vi "B_WriteAttribute.vi"(0 "reference in":refnum<class "BaseTemplate.lvclass">, 5 "error in (no error)":errorcluster) -> (14 "reference out":refnum<class "BaseTemplate.lvclass">, 19 "error out":errorcluster)   [LabVIEW 2020, in "BaseTemplate.lvclass"]
uses:
  <resource>/Framework/Providers/Open_GDS/ClassProviders/Provider_EndevoGOOP300/Templates/BaseTemplate/BaseTemplate.lvclass
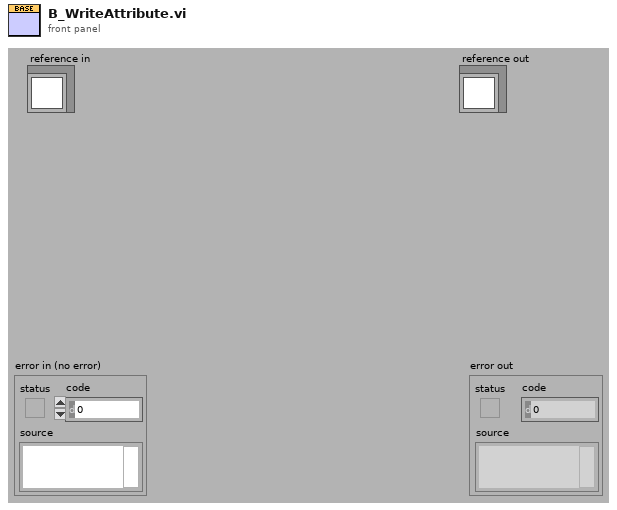
[diagram p1: front panel]
types:
  T1 = typedef "BaseTemplate.lvclass/ObjectAttributes.ctl" = cluster{"Attribute1":dbl}
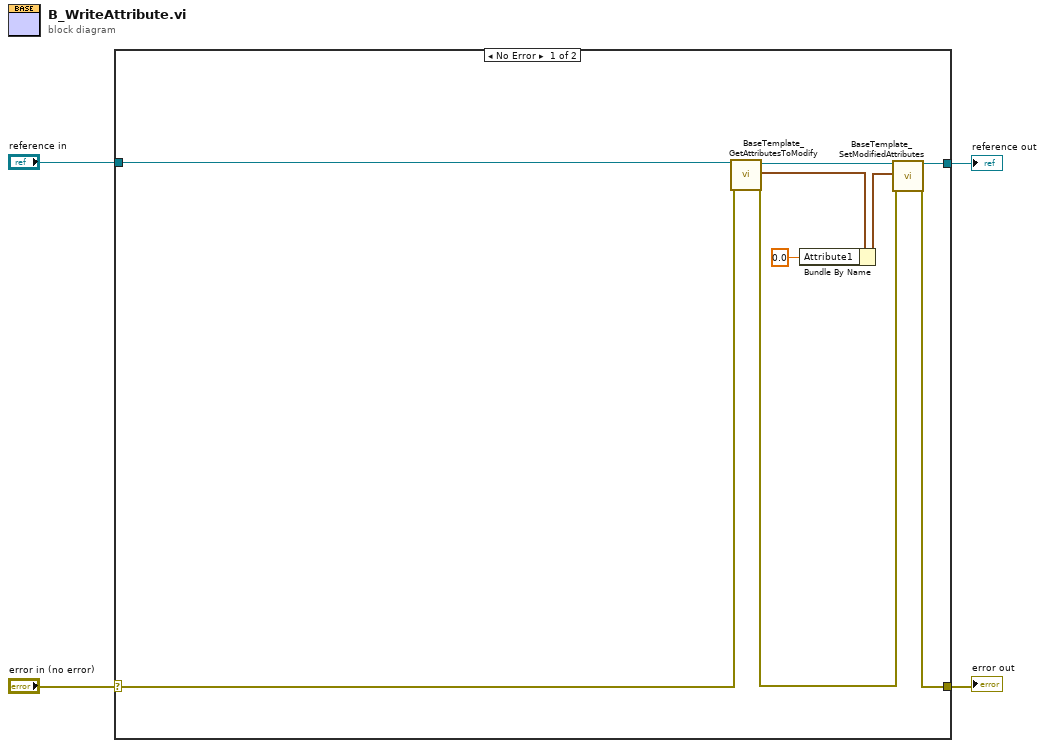
[diagram p0: block diagram]
diagram:
  n1 = case shown="No Error" "error in (no error)" {
    selector: "error in (no error)" -> [w8 w15]
    tunnel: [w10 w15] -> w3
    tunnel: [w7 w14] -> w1
    tunnel: "reference in" -> [w9 w14]
    frame No Error {
      n2 = call <resource>:"BaseTemplate_GetAttributesToModify.vi"("reference in"=w9, "error in (no error)"=w8) -> ("reference out"=w11:refnum<class "BaseTemplate.lvclass">, "Attributes"=w13:T1, "error out"=w5:errorcluster)  [unwired: 14 in, 1 out]
      n3 = Bundle By Name(cluster=w13, "Attribute1"=0.0) -> (w12:T1)
      n4 = call <resource>:"BaseTemplate_SetModifiedAttributes.vi"("reference in"=w11, "Attributes"=w12, "error in (no error)"=w5) -> ("reference out"=w7:refnum<class "BaseTemplate.lvclass">, "error out"=w10:errorcluster)  [unwired: 15 in]
    }
    frame Error {
    }
  }
  "error out" <- w3
  "reference out" <- w1
